vi "ImagerForFlowbit2.vi"() -> ()   [LabVIEW 2011]
uses:
  <vilib>/vision/Image Controls.llb/IMAQ Image.ctl
  <vilib>/Platform/TimedLoop/XDataNode/timing_clust.ctl
  <vilib>/Platform/TimedLoop/XDataNode/nitl_modes.ctl
  <vilib>/Platform/TimedLoop/XDataNode/wakeup.ctl
  <vilib>/Analysis/1siggen.llb/Riffle Array (I32).vi
  <vilib>/Platform/TimedLoop/XDataNode/XDataNode.xnode
  <vilib>/Analysis/NI_AALBase.lvlib
  <vilib>/vision/NI_Vision_Development_Module.lvlib
  <vilib>/Platform/TimedLoop/XDataNode/XDNodeRunTimeDep.lvlib
panel:
  out "队列输出":refnum<queue>
  out "OnlineMap Array":T1[](array[typedef])
  out "DR/R array":T1[](array[typedef])
  out "停止循环":bool
  in  "Stimuli":i32=5
  in  "FrameHeight":i32=576
  in  "FrameWidth":i32=704
  in  "选项卡控件":enum32{"前面板", "参数设置", "OnLineMap"}(tab)
  out "log":string
  out "Stim_ID":i32(listbox)=1
  in  "开始/暂停":bool=TRUE
  in  "停止":bool
  out "重排的 Stim ID":i32[](array[numeric]) caption="重排的{X}"
  out "重排的 Stim ID Index":i32[](array[numeric]) caption="重排的索引"
  out "block":i32
  out "队列中元素数量":i32
  out "Image 2":T1(plugin-control)
  in  "热图":bool
  out "循环持续时间":i64
  out "Recording":bool
  in  "FramesPerStim(100Hz)":i32=16
  in  "Blk目录":path=path "D:/Expt/test"
  in  "文件名":string="G4_E05"
  in  "TimeForPrepare(ms)":u32=1000
  in  "stim ID":u8[](array[numeric])=[0, 2, 4, 6, 8]
  in  "blk总数":i32=500
  in  "stim protocol":T2(array[ring])=[enum."prep stim", enum."wait respirator", enum."show stim", enum."recording data", enum."Blank stim", enum."write data", enum."DR/R", enum."ISI"]
  in  "blank stim":u8
  in  "wait（ms）":u32=10
  in  "ISI（ms）":u32=8000
  in  "FrameBin":i32=25
  in  "datatype":u16(ring)=13 items=["U8"=11, "I16"=12, "U32"=13, "SGL"=14]
  in  "OnlineMap":cluster{"数组 1":i32[], "数组 2":i32[]}[](array[cluster])=[{"数组 1"=[2], "数组 2"=[6]}, {"数组 1"=[4], "数组 2"=[8]}, {"数组 1"=[2, 6], "数组 2"=[4, 8]}, {"数组 1"=[2, 4, 6, 8], "数组 2"=[0]}, {"数组 1"=[2, 4], "数组 2"=[6, 8]}]
  in  "DR/R parameter":T3={"frame_zero_0"=0, "frame_zero_1"=1, "frame_0"=3, "frame_1"=15}
  # "÷"
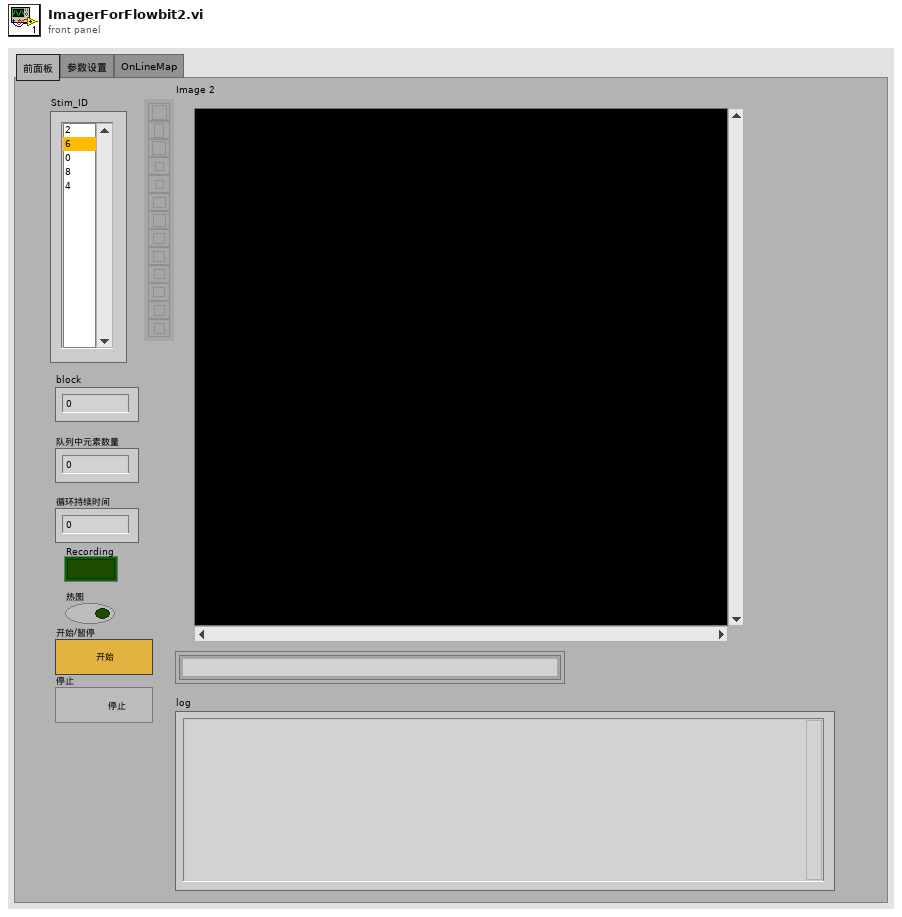
[diagram p1: front panel]
types:
  T1 = typedef "IMAQ Image.ctl" = refnum<image>
  T2 = enum16{"wait", "prep stim", "show stim", "wait respirator", "recording data", "write data", "Blank stim", "wait heart", "ISI", "DR/R", "wait calibrate"}[]
  T3 = cluster{"frame_zero_0":i32, "frame_zero_1":i32, "frame_0":i32, "frame_1":i32}
  T4 = typedef "Image Type" = u32
  T5 = enum16{"Disable External Trigger", "Enable External Trigger"}
  T6 = enum32{"Auto Detect", "RoadRunner", "Raven", "R64"}
  T7 = enum16{"open", "replace", "create", "open or create", "replace or create", "replace or create with confirmation"}
  T8 = enum16{"big-endian, network order", "native, host order", "little-endian"}
  T9 = cluster{"Mean Value":sgl, "Standard Variation":sgl, "Minimal Value":sgl, "Maximal Value":sgl, "Area (calibrated)":sgl, "Area (pixels)":u32, "%":sgl, "Calibration Valid":bool}
  T10 = typedef "XDNodeRunTimeDep.lvlib/timing_clust.ctl" = cluster{"Expected End [f-1]":u64, "Actual End [f-1]":u64, "Finished Late? [f-1]":bool, "Expected End [i-1]":u64, "Actual End [i-1]":u64, "Finished Late? [i-1]":bool, "Expected Start [i]":u64, "Actual Start [i]":u64, "Expected Start [f]":u64, "Actual Start [f]":u64, "Source Name":string, "Structure Name":string, "Period":i64, "Deadline":i64, "Offset":i64, "Start":i64, "Priority":i32, "Timeout":i32, "Mode":T11, "Wakeup Reason":T12, "Error":errorcluster, "Source Type":string, "Secondary Source Type":string, "Global End Time":u64, "Global Start Time":u64, "Frame Duration":u64, "Iteration Duration":u64, "Assigned CPU":i32, "I/O Scan Engine Mode":u32}
  T11 = typedef "XDNodeRunTimeDep.lvlib/nitl_modes.ctl" = enum32{"No Change", "Process missed periods, maintain original phase", "Discard missed periods, maintain original phase", "Process missed periods, ignore original phase", "Discard missed periods, ignore original phase"}
  T12 = typedef "XDNodeRunTimeDep.lvlib/wakeup.ctl" = enum32{"Normal", "Aborted", "Asynchronous wakeup", "Timing source error", "Timed loop error", "Timeout"}
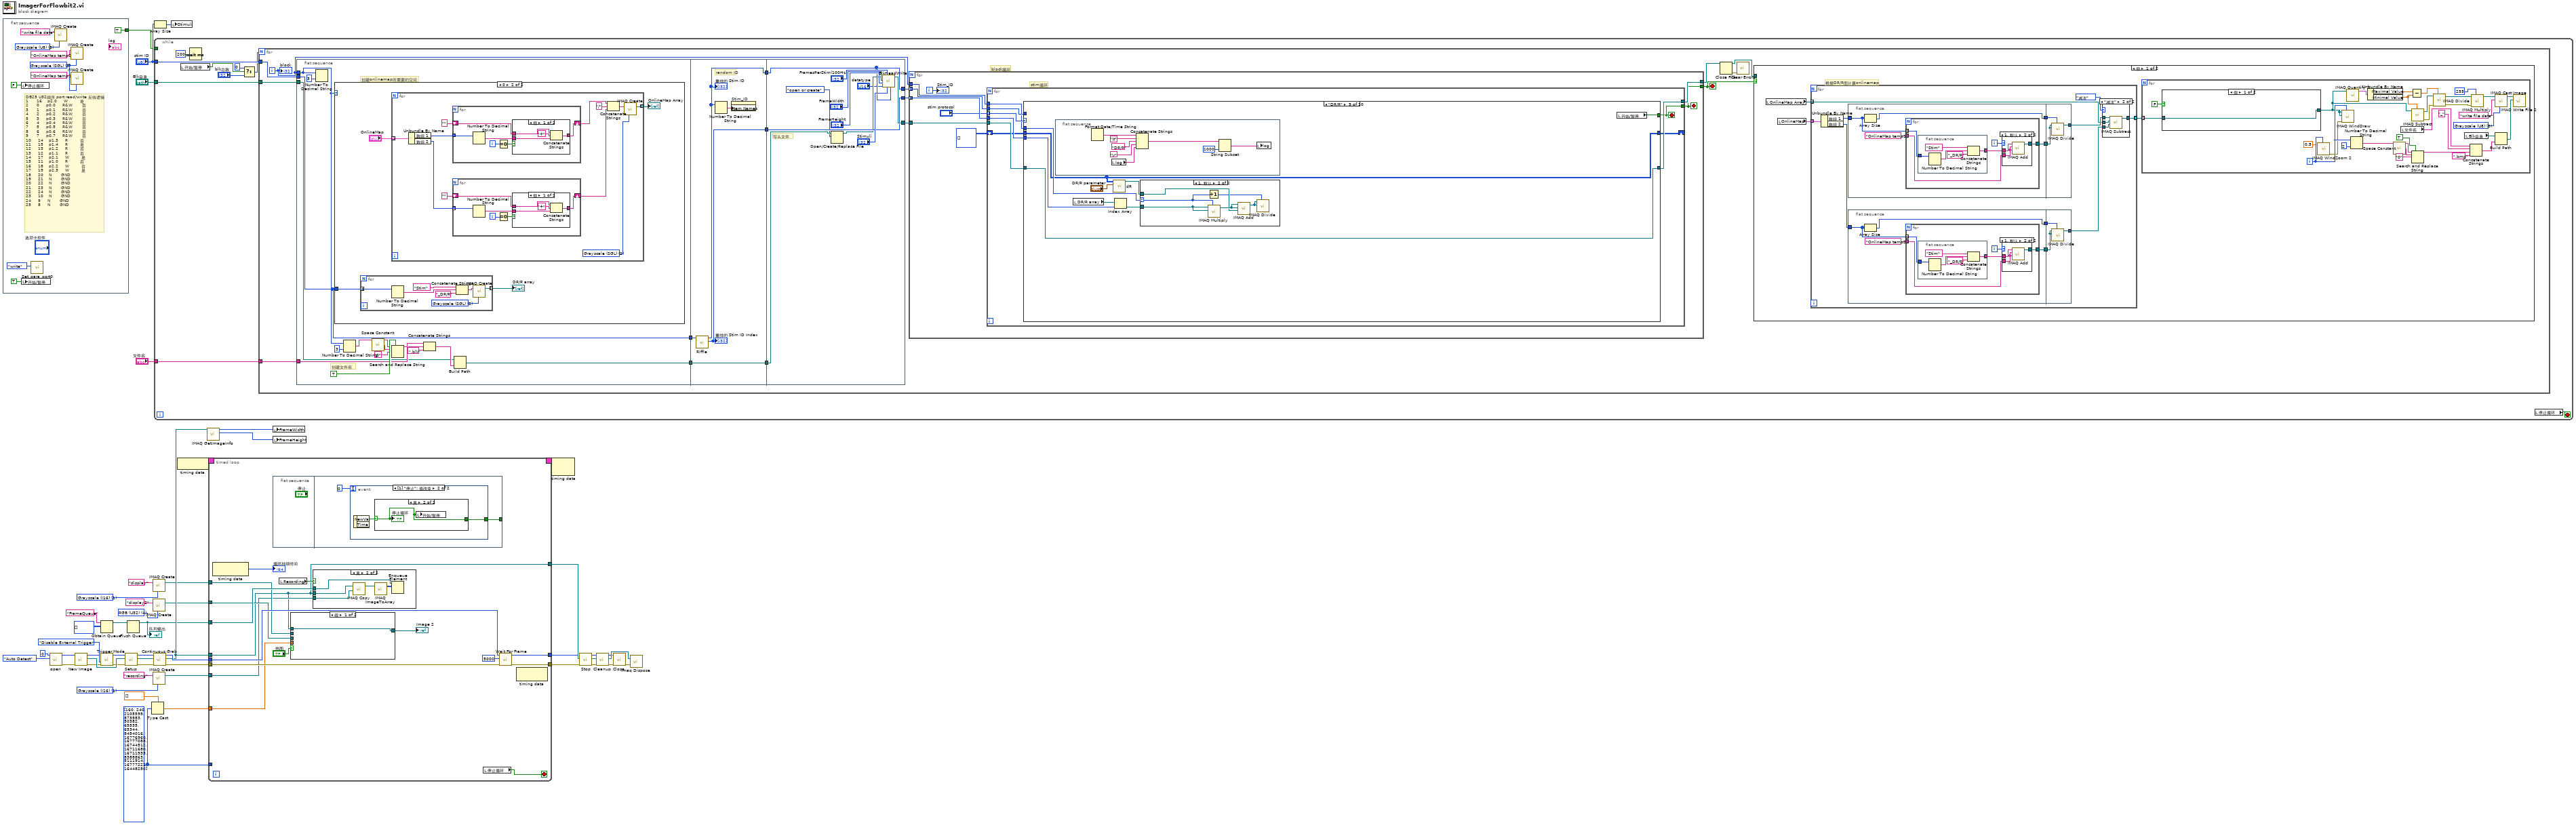
[diagram p0: block diagram]
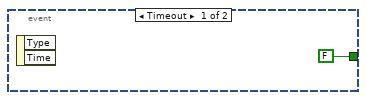
[diagram p2: hidden frame]
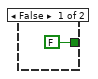
[diagram p3: hidden frame]
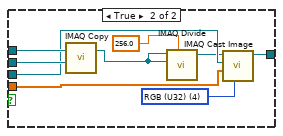
[diagram p4: hidden frame]
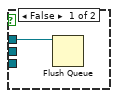
[diagram p5: hidden frame]
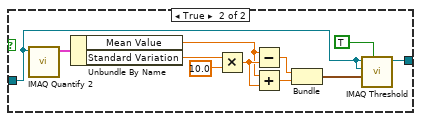
[diagram p6: hidden frame]
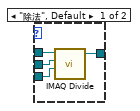
[diagram p7: hidden frame]
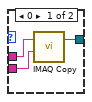
[diagram p8: hidden frame]
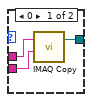
[diagram p9: hidden frame]
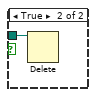
[diagram p10: hidden frame]
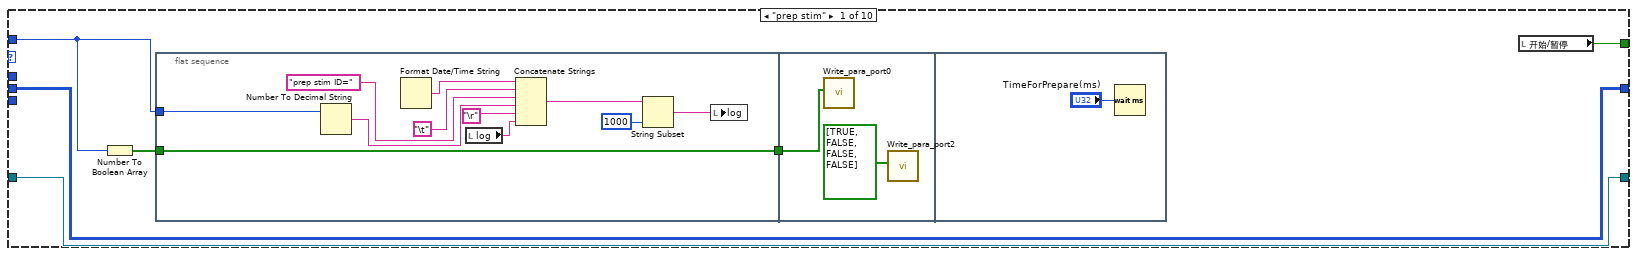
[diagram p14: hidden frame]
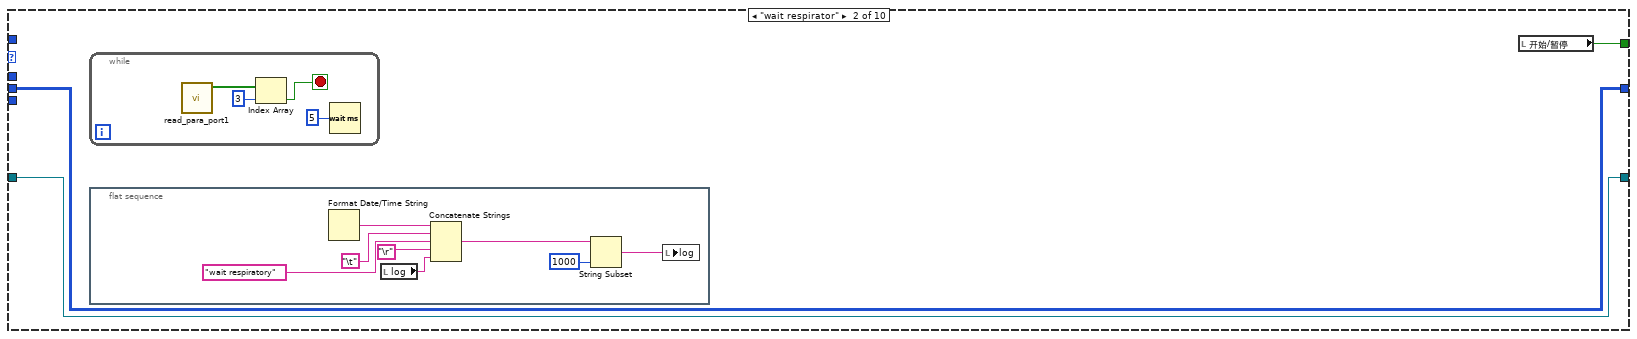
[diagram p15: hidden frame]
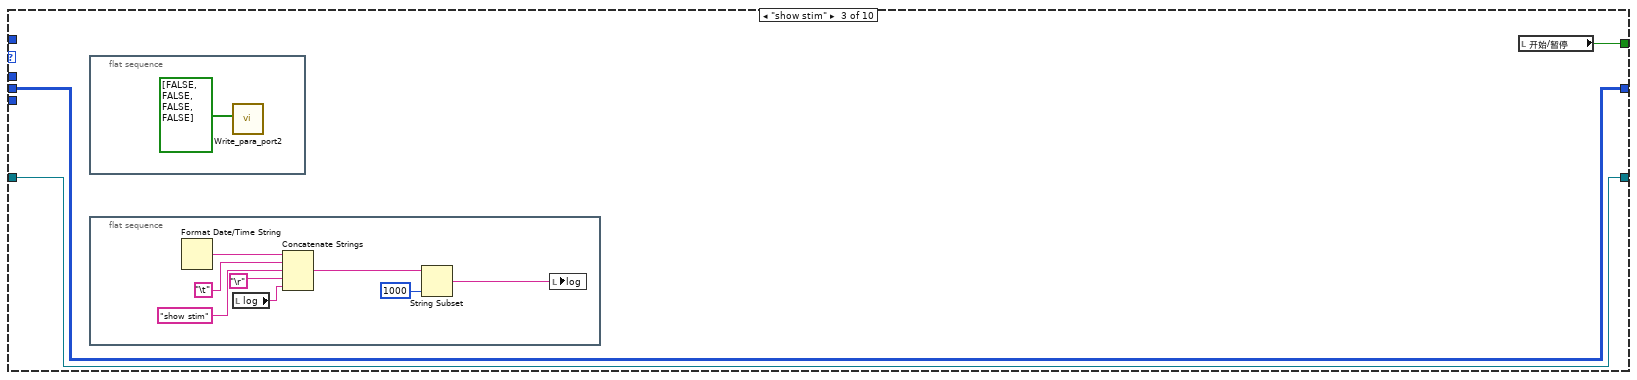
[diagram p16: hidden frame]
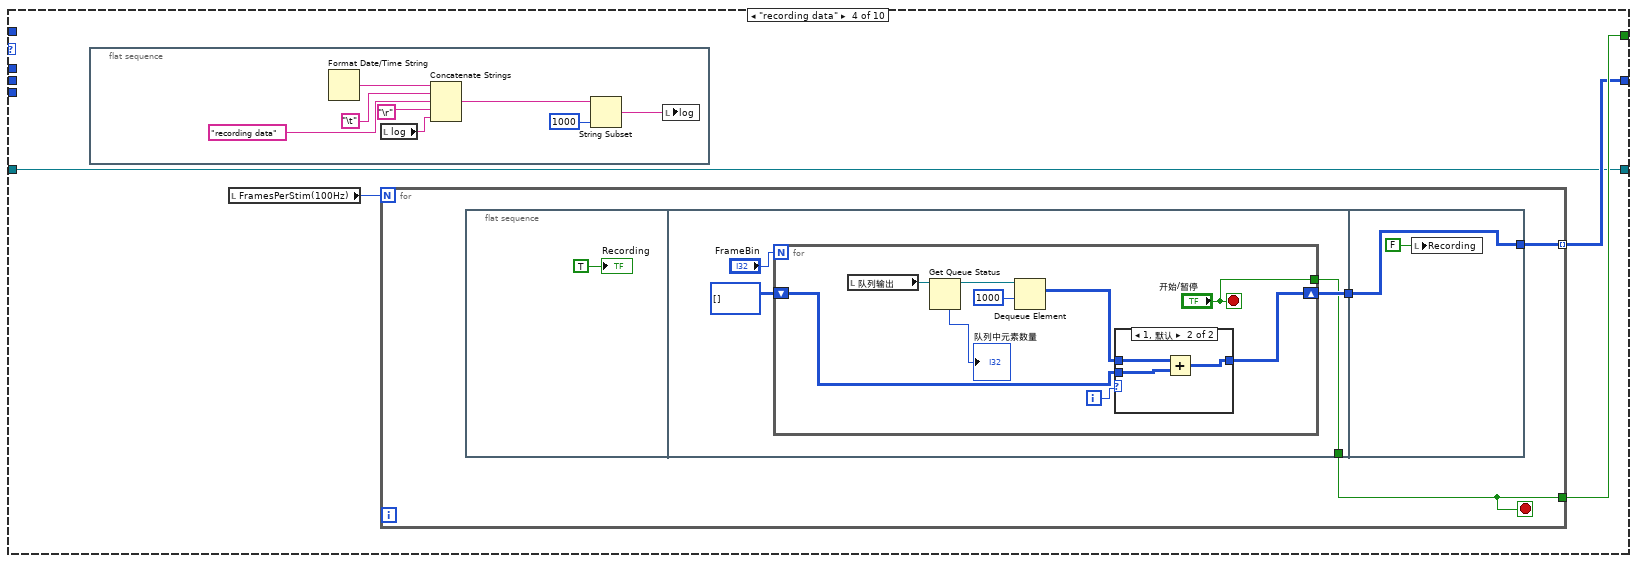
[diagram p17: hidden frame]
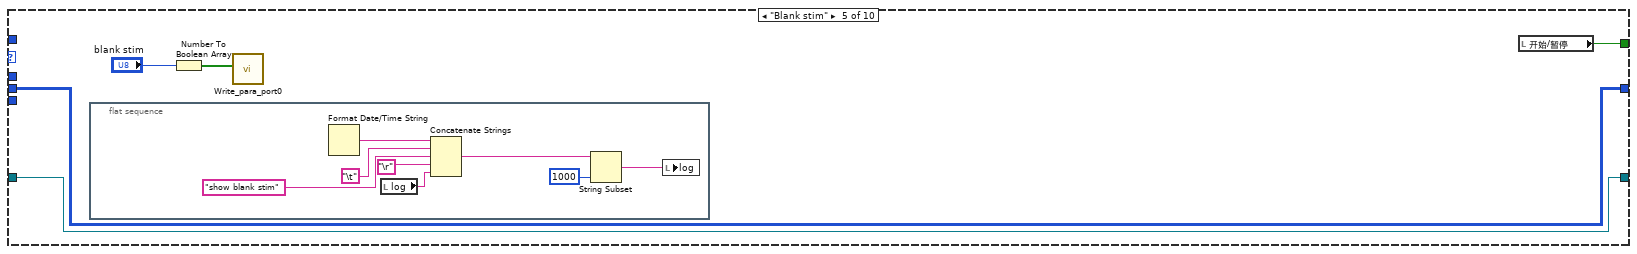
[diagram p19: hidden frame]
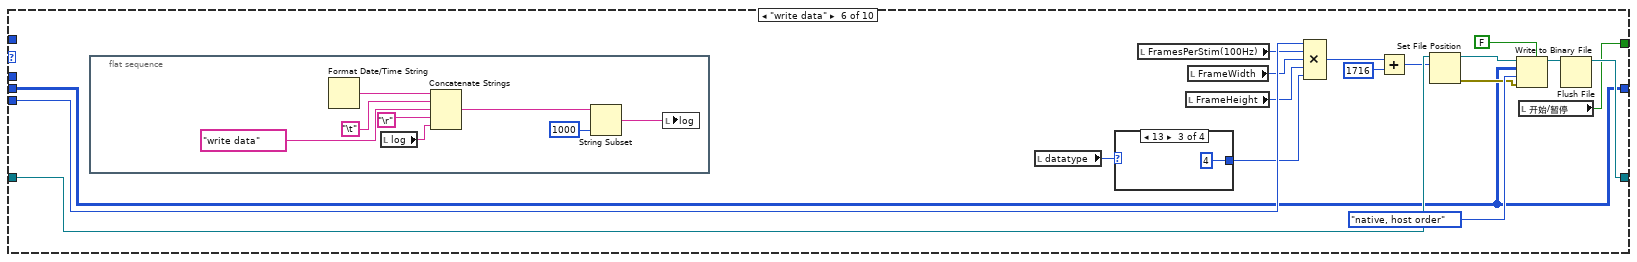
[diagram p20: hidden frame]
diagram:
  w12 = T4 4 items=["Grayscale (U8)", "Grayscale (I16)", "Grayscale (SGL)", "Complex (CSG)", "RGB (U32)", "HSL (U32)", "RGB (U64)", "Grayscale (U16)"] ("Image Type")
  w10 = u32[] [160, 240, 2105599, 873983, 50382, 65535, 65344, 8454016, 16776960, 16777088, 16744512, 16711680, 16711935, 8388863, 5111914, 16777222, 16448250] ("数组")
  w16 = T4 1 items=["Grayscale (U8)", "Grayscale (I16)", "Grayscale (SGL)", "Complex (CSG)", "RGB (U32)", "HSL (U32)", "RGB (U64)", "Grayscale (U16)"] ("Image Type")
  w18 = T4 1 items=["Grayscale (U8)", "Grayscale (I16)", "Grayscale (SGL)", "Complex (CSG)", "RGB (U32)", "HSL (U32)", "RGB (U64)", "Grayscale (U16)"] ("Image Type")
  n1 = flat-sequence {
    tunnel: [TRUE ("Zoom to Fit Mode")] -> w1
    frame #0 {
      w53 = T4 0 items=["Grayscale (U8)", "Grayscale (I16)", "Grayscale (SGL)", "Complex (CSG)", "RGB (U32)", "HSL (U32)", "RGB (U64)", "Grayscale (U16)"] ("Image Type")
      w56 = T4 2 items=["Grayscale (U8)", "Grayscale (I16)", "Grayscale (SGL)", "Complex (CSG)", "RGB (U32)", "HSL (U32)", "RGB (U64)", "Grayscale (U16)"] ("Image Type")
      # "DB25\tU32顺序\tport\tread/write\t反转逻辑\n1\t     16\t   p2.0    \tW\t        是\n2\t     0    \tp0.0\t   \tR&W\t      否\n3\t     1\t\t   p0.1\t   \tR&W      \t否\n4\t\t    2\t   \tp0.2   \t\tR&W      \t否\n5\t\t    3\t\t   p0.3   \t\tR&W\t      否\n6\t\t    4\t   \tp0.4   \t\tR&W      \t否\n7\t\t    5\t   \tp0.5   \t\tR&W      \t否\n8\t\t    6\t   \tp0.6\t   \tR&W      \t否\n9\t    \t7\t   \tp0.7\t   \tR&W\t      否\n10\t    14   \tp1.3   \t\tR        \t否\n11\t   \t15   \tp1.4   \t\tR        \t是\n12\t   \t13   \tp1.2\t   \tR        \t否\n13    \t12   \tp1.1\t   \tR        \t否\n14     17   \tp2.1\t   \tW        \t是\n15    \t11   \tp1.0   \t\tR\t        否\n16    \t18   \tp2.2   \t\tW        \t否\n17    \t19\t   p2.3   \t\tW\t        是\n18    \t20   \tN   \t  \tGND\t\n19    \t21   \tN   \t  \tGND\t\n20\t    22\t   N\t  \t  \tGND\t\n21\t    23\t   N  \t  \t\tGND\t\n22\t    24\t   N  \t  \t\tGND\t\n23    \t10   \tN  \t  \t\tGND\t\n24    \t9\t    N  \t  \t\tGND\t\n25\t    8    \tN  \t  \t\tGND"
      n2 = local write "停止循环"(FALSE ("开始/暂停")) -> ()
      n3 = local write "开始/暂停"(TRUE ("开始/暂停")) -> ()
      n4 = call "Set_para_port0.vi"("R or W"=enum16{"read", "write"}."write") -> ()  [unwired: 9 in, 2 out]
      n5 = call "IMAQ Create"("Image Name"="write file data", "Image Type"=w53) -> ()  [unwired: 3 in, 2 out]
      n6 = call "IMAQ Create"("Image Name"="OnlineMap temp2", "Image Type"=w56) -> ()  [unwired: 3 in, 2 out]
      n7 = call "IMAQ Create"("Image Name"="OnlineMap temp1", "Image Type"=w56) -> ()  [unwired: 3 in, 2 out]
    }
  }
  n8 = call <vilib>:"open.vi"("Board Type"=T6."Auto Detect", "Board Number"=u32 0) -> ("error out"=w34:errorcluster, "RefBrdOut"=w29:u32)  [unwired: 2 in, 5 out]
  n9 = call <vilib>:"New Image.vi"("RefBrdIn"=w29, "error in"=w34) -> ("RefBrdOut"=w28:u32, "Image"=w43:T1, "error out"=w35:errorcluster)  [unwired: 6 in]
  n10 = Obtain Queue(name (unnamed)="FrameQueue" ("名称（未命名）"), element data type=i16[][] []) -> (queue out=w5:refnum<queue>)  [unwired: 3 in, 2 out]
  n11 = call <vilib>:"Trigger Mode.vi"("RefBrdIn"=w28, "Trigger Mode"=T5."Disable External Trigger", "error in (no error)"=w35) -> ("RefBrdOut"=w27:u32, "error out"=w36:errorcluster)  [unwired: 6 in]
  n12 = call <vilib>:"Setup.vi"("error in"=w36, "Image In"=w43, "RefBrdIn"=w27) -> ("error out"=w31:errorcluster, "Image"=w32:T1, "RefBrdOut"=w26:u32)  [unwired: 6 in]
  n13 = Flush Queue(queue=w5) -> (queue out=w4:refnum<queue>)  [unwired: 1 in, 2 out]
  "队列输出" <- w4
  n14 = Type Cast(type=sgl[] [] ("单精度浮点"), x=w10) -> (*(type *) &x=w8:sgl[])
  n15 = call "IMAQ Create"("Image Name"="display", "Image Type"=w16) -> ("New Image"=w14:T1)  [unwired: 3 in, 1 out]
  n16 = call "IMAQ Create"("Image Name"="display2", "Image Type"=w12) -> ("New Image"=w11:T1)  [unwired: 3 in, 1 out]
  n17 = call "IMAQ Create"("Image Name"="recording", "Image Type"=w18) -> ("New Image"=w20:T1)  [unwired: 3 in, 1 out]
  n18 = call <vilib>:"Continuous Grab.vi"("error in (no error)"=w31, "Image In"=w32, "RefBrdIn"=w26) -> ("error out"=w30:errorcluster, "Image"=w17:T1, "RefBrdOut"=w25:u32)  [unwired: 6 in]
  n19 = Array Size(array="stim ID") -> (size(s)=w49:i32)
  n20 = while {
    tunnel: "stim ID" -> [w69]
    tunnel: "文件名" -> [w68]
    tunnel: "Blk目录" -> [w67]
    tunnel: w1 -> [_]
    stop <- w65 stop-if-true
    n21 = local read "开始/暂停"() -> (w64:bool)
    n22 = Wait (ms)(milliseconds to wait=u32 200 ("等待时间（毫秒）")) -> ()  [unwired: 1 out]
    n23 = Select(t=0, s=w64, f="blk总数") -> (s? t:f=w61:i32)
    n24 = for {
      N: w61 -> [_]
      tunnel: w69 -> [w73]
      tunnel: w68 -> [w85]
      tunnel: w67 -> [w84]
      i -> [w74]
      stop <- w76 stop-if-true
      # "block循环"
      n25 = flat-sequence {
        tunnel: [w201] -> w82
        tunnel: [w200] -> w72
        tunnel: w74 -> [w199]
        tunnel: w85 -> [w206]
        tunnel: w84 -> [w202]
        tunnel: w73 -> [w200]
        tunnel: w82 -> [w261]
        tunnel: [w261] -> w81
        tunnel: [w259] -> w80
        tunnel: w72 -> [w258]
        tunnel: [w257] -> w71
        tunnel: w81 -> [w265]
        tunnel: [w268] -> w83
        tunnel: w80 -> [w267]
        tunnel: [w267] -> w79
        tunnel: w71 -> [w266]
        tunnel: [w266] -> w70
        frame #0 {
          # "创建onlinemap所需要的空间"
          # "创建文件名"
          n26 = Number To Decimal String(number=w199, width (-)=i16 3 ("宽度(-)")) -> ()  [unwired: 1 out]
          n27 = case shown="0" w199 {
            tunnel: w200 -> [_ w216]
            frame 1, Default {
            }
            frame 0 {
              n28 = for {
                tunnel: w216 -> [w253] mode=indexing
                tunnel: [w250] -> w215 mode=indexing
                w256 = T4 2 items=["Grayscale (U8)", "Grayscale (I16)", "Grayscale (SGL)", "Complex (CSG)", "RGB (U32)", "HSL (U32)", "RGB (U64)", "Grayscale (U16)"] ("Image Type")
                n29 = Number To Decimal String(number=w253) -> (decimal integer string=w254:string)  [unwired: 1 in]
                n30 = Concatenate Strings("Stim", w254, "_DR/R" ("字符串")) -> (w251:string)
                n31 = call "IMAQ Create"("Image Name"=w251, "Image Type"=w256) -> ("New Image"=w250:T1)  [unwired: 3 in, 1 out]
              }
              "DR/R array" <- w215
              n32 = for {
                tunnel: "OnlineMap" -> [w227] mode=indexing
                tunnel: [w217] -> w213 mode=indexing
                w225 = T4 2 items=["Grayscale (U8)", "Grayscale (I16)", "Grayscale (SGL)", "Complex (CSG)", "RGB (U32)", "HSL (U32)", "RGB (U64)", "Grayscale (U16)"] ("Image Type")
                n33 = Unbundle By Name(w227) -> ("数组 1"=w226:i32[], "数组 2"=w222:i32[])
                n34 = for {
                  tunnel: w226 -> [w242] mode=indexing
                  shift-right: [w240] -> w223
                  shift-left: "" -> [w239]
                  i -> [w244]
                  n35 = Number To Decimal String(number=w242) -> (decimal integer string=w241:string)  [unwired: 1 in]
                  n36 = Equal To 0?(x=w244) -> (x = 0?=w243:bool)
                  n37 = case shown="假" w243 {
                    tunnel: w241 -> [w245 w249]
                    tunnel: [w248 w249] -> w240
                    tunnel: w239 -> [w247 _]
                    frame False {
                      n38 = Concatenate Strings(w247, "+" ("字符串"), w245) -> (w248:string)
                    }
                    frame True {
                    }
                  }
                }
                n39 = for {
                  tunnel: w222 -> [w231] mode=indexing
                  shift-right: [w229] -> w220
                  shift-left: "" -> [w228]
                  i -> [w233]
                  n40 = Number To Decimal String(number=w231) -> (decimal integer string=w230:string)  [unwired: 1 in]
                  n41 = Equal To 0?(x=w233) -> (x = 0?=w232:bool)
                  n42 = case shown="假" w232 {
                    tunnel: w230 -> [w234 w238]
                    tunnel: [w237 w238] -> w229
                    tunnel: w228 -> [w236 _]
                    frame False {
                      n43 = Concatenate Strings(w236, "+" ("字符串"), w234) -> (w237:string)
                    }
                    frame True {
                    }
                  }
                }
                n44 = Concatenate Strings(w223, "/" ("字符串"), w220) -> (w218:string)
                n45 = call "IMAQ Create"("Image Name"=w218, "Image Type"=w225) -> ("New Image"=w217:T1)  [unwired: 3 in, 1 out]
              }
              "OnlineMap Array" <- w213
            }
          }
          n46 = Number To Decimal String(number=w199, width (-)=i16 3 ("宽度(-)")) -> (decimal integer string=w208:string)
          n47 = call <vilib>:"Space Constant.vi"() -> ("String"=w209:string)
          n48 = Search and Replace String(replace all?=TRUE ("替换全部？(F)"), input string=w208, search string=w209, replace string="0" ("替换字符串(\"\")")) -> (result string=w205:string)  [unwired: 4 in, 3 out]
          n49 = Concatenate Strings(w206, w205, ".blk" ("字符串")) -> (w203:string)
          n50 = Build Path(base path=w202, name or relative path=w203) -> (appended path=w201:path)
        }
        frame #1 {
          # "random ID"
          n51 = call-poly <vilib>:"Riffle.vi"("X"=w258) -> ("Riffled Index"=w257:i32[], "Riffled {X}"=w259:i32[])  [unwired: 8 in, 1 out]
          "重排的 Stim ID Index" <- w257
          "重排的 Stim ID" <- w259
          n52 = Number To Decimal String(number=w259) -> (decimal integer string=w260:string[])  [unwired: 1 in]
          n53 = property on="Stim_ID" class="LstBox (严格)"("Item Names"=w260) -> ()  [unwired: 2 in, 2 out]
        }
        frame #2 {
          # "写头文件"
          n54 = Open/Create/Replace File(file path (use dialog)=w265, operation (0:open)=T7."open or create" ("操作(0:open)")) -> (refnum out=w263:refnum<file>)  [unwired: 4 in, 2 out]
          n55 = call "BlkHeadWrite.vi"("SequenceOfID"=w267, "Stimuli"="Stimuli", "FramesPerStim"="FramesPerStim(100Hz)", "datatype"="datatype", "FrameHeight"="FrameHeight", "FrameWidth"="FrameWidth", "BlkFile"=w263) -> ("引用句柄输出"=w268:refnum<file>)  [unwired: 4 in]
        }
      }
      n56 = for {
        tunnel: w83 -> [w281]
        tunnel: [w279] -> w77
        tunnel: w70 -> [w280] mode=indexing
        tunnel: w79 -> [w278] mode=indexing
        tunnel: [w277] -> w76
        tunnel: w74 -> [w273]
        i -> [w276]
        stop <- w277 stop-if-true
        # "stim循环"
        n57 = for {
          tunnel: w280 -> [w289]
          tunnel: w278 -> [w287]
          tunnel: [w283] -> w277
          shift-right: [w286] -> _
          shift-left: u32[][][] [] ("初始化的数组") -> [w285]
          tunnel: "stim protocol" -> [w284] mode=indexing
          tunnel: w281 -> [w290]
          tunnel: [w288] -> w279
          tunnel: w273 -> [w282]
          stop <- w283 stop-if-true
          n58 = case shown="\"DR/R\"" w284 {
            tunnel: w290 -> [w293 w311 w326 w338 w373 w403 w417 w432 w452 w470]
            tunnel: w289 -> [_ _ _ _ _ w402 _ _ w450 _]
            tunnel: [w293 w311 w326 w338 w373 w390 w417 w432 w452 w470] -> w288
            tunnel: w287 -> [w291 _ _ _ _ _ _ _ _ _]
            tunnel: [w294 w312 w327 w340 w374 w388 w418 w433 w451 w471] -> w283
            tunnel: [w295 w313 w328 w339 w375 w389 w419 w434 w445 w472] -> w286
            tunnel: w285 -> [w295 w313 w328 _ w375 w389 w419 w434 w445 w472]
            tunnel: w282 -> [_ _ _ _ _ _ _ _ w449 _]
            frame "prep stim" {
              n59 = Number To Boolean Array(number=w291) -> (Boolean array=w296:bool[])
              n60 = flat-sequence {
                tunnel: w296 -> [w307]
                tunnel: [w307] -> w292
                tunnel: w291 -> [w306]
                tunnel: w292 -> [w309]
                frame #0 {
                  n61 = Number To Decimal String(number=w306) -> (decimal integer string=w303:string)  [unwired: 1 in]
                  n62 = Format Date/Time String() -> (date/time string=w305:string)  [unwired: 3 in]
                  n63 = local read "log"() -> (w299:string)
                  n64 = Concatenate Strings(w305, "\t", "prep stim ID=" ("字符串"), w303, "\r", w299) -> (w301:string)
                  n65 = String Subset(string=w301, length (rest)=1000 ("y")) -> (substring=w300:string)  [unwired: 1 in]
                  n66 = local write "log"(w300) -> ()
                }
                frame #1 {
                  n67 = call "Write_para_port0.vi"("port0（8元素）"=w309) -> ()  [unwired: 10 in, 1 out]
                  n68 = call "Write_para_port2.vi"("port2（4元素）"=bool[] [TRUE, FALSE, FALSE, FALSE] ("port2")) -> ()  [unwired: 10 in, 1 out]
                }
                frame #2 {
                  n69 = Wait (ms)(milliseconds to wait="TimeForPrepare(ms)") -> ()  [unwired: 1 out]
                }
              }
              n70 = local read "开始/暂停"() -> (w294:bool)
            }
            frame "wait respirator" {
              n71 = while {
                stop <- w323 stop-if-true
                n72 = call "read_para_port1.vi"() -> ("port1（5元素）"=w325:bool[])  [unwired: 10 in, 1 out]
                n73 = Index Array(array=w325, index=3 ("索引")) -> (element=w323:bool)
                n74 = Wait (ms)(milliseconds to wait=u32 5 ("等待时间（毫秒）")) -> ()  [unwired: 1 out]
              }
              n75 = flat-sequence {
                frame #0 {
                  n76 = Format Date/Time String() -> (date/time string=w321:string)  [unwired: 3 in]
                  n77 = local read "log"() -> (w316:string)
                  n78 = Concatenate Strings(w321, "\t", "wait respiratory" ("字符串"), "\r", w316) -> (w318:string)
                  n79 = String Subset(string=w318, length (rest)=1000 ("y")) -> (substring=w317:string)  [unwired: 1 in]
                  n80 = local write "log"(w317) -> ()
                }
              }
              n81 = local read "开始/暂停"() -> (w312:bool)
            }
            frame "show stim" {
              n82 = flat-sequence {
                frame #0 {
                  n83 = call "Write_para_port2.vi"("port2（4元素）"=bool[] [FALSE, FALSE, FALSE, FALSE] ("port2")) -> ()  [unwired: 10 in, 1 out]
                }
              }
              n84 = flat-sequence {
                frame #0 {
                  n85 = Format Date/Time String() -> (date/time string=w336:string)  [unwired: 3 in]
                  n86 = local read "log"() -> (w331:string)
                  n87 = Concatenate Strings(w336, "\t", "show stim" ("字符串"), "\r", w331) -> (w333:string)
                  n88 = String Subset(string=w333, length (rest)=1000 ("y")) -> (substring=w332:string)  [unwired: 1 in]
                  n89 = local write "log"(w332) -> ()
                }
              }
              n90 = local read "开始/暂停"() -> (w327:bool)
            }
            frame "recording data" {
              n91 = flat-sequence {
                frame #0 {
                  n92 = Format Date/Time String() -> (date/time string=w349:string)  [unwired: 3 in]
                  n93 = local read "log"() -> (w344:string)
                  n94 = Concatenate Strings(w349, "\t", "recording data" ("字符串"), "\r", w344) -> (w346:string)
                  n95 = String Subset(string=w346, length (rest)=1000 ("y")) -> (substring=w345:string)  [unwired: 1 in]
                  n96 = local write "log"(w345) -> ()
                }
              }
              n97 = local read "FramesPerStim(100Hz)"() -> (w341:i32)
              n98 = for {
                N: w341 -> [_]
                tunnel: [w350] -> w339 mode=indexing
                tunnel: [w352] -> w340
                stop <- w352 stop-if-true
                n99 = flat-sequence {
                  tunnel: [w354] -> w352
                  tunnel: [w356] -> w351
                  tunnel: [w372] -> w350
                  tunnel: w351 -> [w372]
                  frame #0 {
                    "Recording" <- TRUE ("Recording")
                  }
                  frame #1 {
                    n100 = for {
                      N: "FrameBin" -> [_]
                      shift-right: [w365] -> w356
                      shift-left: u32[][] [] ("初始化的数组") -> [w366]
                      tunnel: ["开始/暂停"] -> w354
                      i -> [w364]
                      stop <- "开始/暂停" stop-if-true
                      n101 = local read "队列输出"() -> (w362:refnum<queue>)
                      n102 = Get Queue Status(queue=w362) -> (queue out=w360:refnum<queue>, # elements in queue=→"队列中元素数量":i32)  [unwired: 2 in, 6 out]
                      n103 = Dequeue Element(queue=w360, timeout in ms (-1)=1000 ("超时毫秒(-1)")) -> (element=w359:i16[][])  [unwired: 1 in, 3 out]
                      n104 = case shown="1, 默认" w364 {
                        tunnel: w359 -> [w367 w370]
                        tunnel: w366 -> [_ w369]
                        tunnel: [w367 w368] -> w365
                        frame 0 {
                        }
                        frame 1, Default {
                          n105 = Add(x=w370, y=w369) -> (x+y=w368:u32[][])
                        }
                      }
                    }
                  }
                  frame #2 {
                    n106 = local write "Recording"(FALSE ("Recording")) -> ()
                  }
                }
              }
            }
            frame "Blank stim" {
              n107 = flat-sequence {
                frame #0 {
                  n108 = Format Date/Time String() -> (date/time string=w385:string)  [unwired: 3 in]
                  n109 = local read "log"() -> (w380:string)
                  n110 = Concatenate Strings(w385, "\t", "show blank stim" ("字符串"), "\r", w380) -> (w382:string)
                  n111 = String Subset(string=w382, length (rest)=1000 ("y")) -> (substring=w381:string)  [unwired: 1 in]
                  n112 = local write "log"(w381) -> ()
                }
              }
              n113 = Number To Boolean Array(number="blank stim") -> (Boolean array=w376:bool[])
              n114 = call "Write_para_port0.vi"("port0（8元素）"=w376) -> ()  [unwired: 10 in, 1 out]
              n115 = local read "开始/暂停"() -> (w374:bool)
            }
            frame "write data" {
              n116 = flat-sequence {
                frame #0 {
                  n117 = Format Date/Time String() -> (date/time string=w415:string)  [unwired: 3 in]
                  n118 = local read "log"() -> (w410:string)
                  n119 = Concatenate Strings(w415, "\t", "write data" ("字符串"), "\r", w410) -> (w412:string)
                  n120 = String Subset(string=w412, length (rest)=1000 ("y")) -> (substring=w411:string)  [unwired: 1 in]
                  n121 = local write "log"(w411) -> ()
                }
              }
              n122 = local read "datatype"() -> (w387:u16)
              n123 = case shown="13" w387 {
                tunnel: [1 2 4 4] -> w386
                frame 11, Default {
                }
                frame 12 {
                }
                frame 13 {
                }
                frame 14 {
                }
              }
              n124 = local read "FramesPerStim(100Hz)"() -> (w394:i32)
              n125 = local read "FrameHeight"() -> (w392:i32)
              n126 = local read "FrameWidth"() -> (w393:i32)
              n127 = Compound Arithmetic op=MULTIPLY(w402, w394, w393, w392, w386) -> (w397:i32)
              n128 = Add(x=w397, y=i64 1716 ("偏移量（字节）（0）")) -> (x+y=w395:i64)
              n129 = Set File Position(offset (in bytes) (0)=w395, refnum=w403) -> (refnum out=w400:refnum<file>, error out=w398:errorcluster)  [unwired: 2 in]
              n130 = Write to Binary File(file (use dialog)=w400, data=w389, error in=w398, 5:FALSE ("预置数组或字符串大小？(T)"), 9:T8."native, host order" ("字节顺序(0:big-endian, network order)")) -> (refnum out=w391:refnum<file>)  [unwired: 1 in, 2 out]
              n131 = local read "开始/暂停"() -> (w388:bool)
              n132 = Flush File(refnum=w391) -> (refnum out=w390:refnum<file>)  [unwired: 1 in, 1 out]
            }
            frame "ISI" {
              n133 = flat-sequence {
                tunnel: "ISI（ms）" -> [w423]
                tunnel: "ISI（ms）" -> [w430]
                frame #0 {
                  n134 = Number To Decimal String(number=w423) -> (decimal integer string=w427:string)  [unwired: 1 in]
                  n135 = Format Date/Time String() -> (date/time string=w429:string)  [unwired: 3 in]
                  n136 = local read "log"() -> (w422:string)
                  n137 = Concatenate Strings(w429, "\t", "ISI(ms)=" ("字符串"), w427, "\r", w422) -> (w425:string)
                  n138 = String Subset(string=w425, length (rest)=1000 ("y")) -> (substring=w424:string)  [unwired: 1 in]
                  n139 = local write "log"(w424) -> ()
                }
                frame #1 {
                  n140 = Wait (ms)(milliseconds to wait=w430) -> ()  [unwired: 1 out]
                }
              }
              n141 = local read "开始/暂停"() -> (w418:bool)
            }
            frame "wait", Default {
              n142 = Wait (ms)(milliseconds to wait="wait（ms）") -> ()  [unwired: 1 out]
              n143 = flat-sequence {
                tunnel: "wait（ms）" -> [w438]
                frame #0 {
                  n144 = Number To Decimal String(number=w438) -> (decimal integer string=w442:string)  [unwired: 1 in]
                  n145 = Format Date/Time String() -> (date/time string=w444:string)  [unwired: 3 in]
                  n146 = local read "log"() -> (w437:string)
                  n147 = Concatenate Strings(w444, "\t", "wait(ms)=" ("字符串"), w442, "\r", w437) -> (w440:string)
                  n148 = String Subset(string=w440, length (rest)=1000 ("y")) -> (substring=w439:string)  [unwired: 1 in]
                  n149 = local write "log"(w439) -> ()
                }
              }
              n150 = local read "开始/暂停"() -> (w433:bool)
            }
            frame "DR/R" {
              n151 = flat-sequence {
                frame #0 {
                  n152 = Format Date/Time String() -> (date/time string=w461:string)  [unwired: 3 in]
                  n153 = local read "log"() -> (w456:string)
                  n154 = Concatenate Strings(w461, "\t", "DR/R" ("字符串"), "\r", w456) -> (w458:string)
                  n155 = String Subset(string=w458, length (rest)=1000 ("y")) -> (substring=w457:string)  [unwired: 1 in]
                  n156 = local write "log"(w457) -> ()
                }
              }
              n157 = local read "DR/R array"() -> (w446:T1[])
              n158 = call "dR.vi"("DR/R parameter"="DR/R parameter", "数组"=w445) -> ("Image Dst Out"=w448:T1)  [unwired: 9 in]
              n159 = Index Array(array=w446, index=w450) -> (element=w447:T1)
              n160 = case shown="1, 默认" w449 {
                selector: w449 -> [_ w466]
                tunnel: w448 -> [w463 w467]
                tunnel: w447 -> [w462 w469]
                frame 0 {
                  n161 = call "IMAQ Copy"("Image Dst"=w462, "Image Src"=w463) -> ()  [unwired: 4 in, 2 out]
                }
                frame 1, Default {
                  n162 = Increment(x=w466) -> (x+1=w465:i32)
                  n163 = call "IMAQ Multiply"("Image Src A"=w469, "Constant"=w466, "Image Dst"=w469) -> ("Image Dst Out"=w468:T1)  [unwired: 4 in, 1 out]
                  n164 = call "IMAQ Add"("Image Src A"=w468, "Image Dst"=w468, "Image Src B"=w467) -> ("Image Dst Out"=w464:T1)  [unwired: 4 in, 1 out]
                  n165 = call "IMAQ Divide"("Image Src A"=w464, "Constant"=w465, "Image Dst"=w464) -> ()  [unwired: 4 in, 2 out]
                }
              }
              n166 = local read "开始/暂停"() -> (w451:bool)
            }
            frame "wait heart" {
              n167 = flat-sequence {
                frame #0 {
                  n168 = Format Date/Time String() -> (date/time string=w480:string)  [unwired: 3 in]
                  n169 = local read "log"() -> (w475:string)
                  n170 = Concatenate Strings(w480, "\t", "wait heart" ("字符串"), "\r", w475) -> (w477:string)
                  n171 = String Subset(string=w477, length (rest)=1000 ("y")) -> (substring=w476:string)  [unwired: 1 in]
                  n172 = local write "log"(w476) -> ()
                }
              }
              n173 = local read "开始/暂停"() -> (w471:bool)
            }
          }
        }
        "Stim_ID" <- w276
      }
      n174 = Close File(refnum=w77) -> (path=w75:path, error out=w78:errorcluster)  [unwired: 1 in]
      n175 = call <vilib>:"Clear Errors.vi"("error in (no error)"=w78) -> ()  [unwired: 6 in, 1 out]
      n176 = case shown="假" w76 {
        tunnel: w75 -> [_ w198]
        frame False {
          # "根据DR/R图计算onlinemap"
          n177 = local read "OnlineMap Array"() -> (w87:T1[])
          n178 = local read "OnlineMap"() -> (w88:cluster{"数组 1":i32[], "数组 2":i32[]}[])
          n179 = for {
            tunnel: w88 -> [w143] mode=indexing
            tunnel: w87 -> [w134] mode=indexing
            tunnel: [w132] -> w86 mode=indexing
            n180 = Unbundle By Name(w143) -> ("数组 1"=w142:i32[], "数组 2"=w137:i32[])
            n181 = flat-sequence {
              tunnel: w142 -> [w177]
              tunnel: [w176] -> w141
              tunnel: [w175] -> w140
              tunnel: w141 -> [w196]
              tunnel: w140 -> [w197]
              tunnel: [w195] -> w136
              frame #0 {
                n182 = Array Size(array=w177) -> (size(s)=w175:i32)
                n183 = for {
                  tunnel: w177 -> [w183] mode=indexing
                  tunnel: "OnlineMap temp1" ("Image Name") -> [w181]
                  tunnel: [w179] -> w176
                  i -> [w180]
                  n184 = flat-sequence {
                    tunnel: w183 -> [w192]
                    tunnel: [w190] -> w182
                    frame #0 {
                      n185 = Number To Decimal String(number=w192) -> (decimal integer string=w193:string)  [unwired: 1 in]
                      n186 = Concatenate Strings("Stim", w193, "_DR/R" ("字符串")) -> (w190:string)
                    }
                  }
                  n187 = case shown="1, 默认" w180 {
                    tunnel: w182 -> [w186 w189]
                    tunnel: w181 -> [w185 w188]
                    tunnel: [w184 w187] -> w179
                    frame 0 {
                      n188 = call "IMAQ Copy"("Image Dst"=w185, "Image Src"=w186) -> ("Image Dst Out"=w184:T1)  [unwired: 4 in, 1 out]
                    }
                    frame 1, Default {
                      n189 = call "IMAQ Add"("Image Src A"=w189, "Image Dst"=w188, "Image Src B"=w188) -> ("Image Dst Out"=w187:T1)  [unwired: 4 in, 1 out]
                    }
                  }
                }
              }
              frame #1 {
                n190 = call "IMAQ Divide"("Image Src A"=w196, "Constant"=w197, "Image Dst"=w196) -> ("Image Dst Out"=w195:T1)  [unwired: 4 in, 1 out]
              }
            }
            n191 = flat-sequence {
              tunnel: w137 -> [w154]
              tunnel: [w153] -> w139
              tunnel: [w152] -> w138
              tunnel: w139 -> [w173]
              tunnel: w138 -> [w174]
              tunnel: [w172] -> w135
              frame #0 {
                n192 = Array Size(array=w154) -> (size(s)=w152:i32)
                n193 = for {
                  tunnel: w154 -> [w160] mode=indexing
                  tunnel: "OnlineMap temp2" ("Image Name") -> [w158]
                  tunnel: [w156] -> w153
                  i -> [w157]
                  n194 = flat-sequence {
                    tunnel: w160 -> [w169]
                    tunnel: [w167] -> w159
                    frame #0 {
                      n195 = Number To Decimal String(number=w169) -> (decimal integer string=w170:string)  [unwired: 1 in]
                      n196 = Concatenate Strings("Stim", w170, "_DR/R" ("字符串")) -> (w167:string)
                    }
                  }
                  n197 = case shown="1, 默认" w157 {
                    tunnel: w159 -> [w163 w166]
                    tunnel: w158 -> [w162 w165]
                    tunnel: [w161 w164] -> w156
                    frame 0 {
                      n198 = call "IMAQ Copy"("Image Dst"=w162, "Image Src"=w163) -> ("Image Dst Out"=w161:T1)  [unwired: 4 in, 1 out]
                    }
                    frame 1, Default {
                      n199 = call "IMAQ Add"("Image Src A"=w166, "Image Dst"=w165, "Image Src B"=w165) -> ("Image Dst Out"=w164:T1)  [unwired: 4 in, 1 out]
                    }
                  }
                }
              }
              frame #1 {
                n200 = call "IMAQ Divide"("Image Src A"=w173, "Constant"=w174, "Image Dst"=w173) -> ("Image Dst Out"=w172:T1)  [unwired: 4 in, 1 out]
              }
            }
            n201 = case shown="\"减法\"" enum16{"除法", "减法"}."减法" {
              tunnel: w136 -> [w147 w151]
              tunnel: w135 -> [w146 w150]
              tunnel: w134 -> [w145 w149]
              tunnel: [w144 w148] -> w132
              frame "除法", Default {
                n202 = call "IMAQ Divide"("Image Src A"=w147, "Image Dst"=w145, "Image Src B"=w146) -> ("Image Dst Out"=w144:T1)  [unwired: 4 in, 1 out]
              }
              frame "减法" {
                n203 = call "IMAQ Subtract"("Image Src A"=w151, "Image Dst"=w149, "Image Src B"=w150) -> ("Image Dst Out"=w148:T1)  [unwired: 4 in, 1 out]
              }
            }
          }
          n204 = for {
            tunnel: w86 -> [w119] mode=indexing
            i -> [w117]
            w103 = T4 0 items=["Grayscale (U8)", "Grayscale (I16)", "Grayscale (SGL)", "Complex (CSG)", "RGB (U32)", "HSL (U32)", "RGB (U64)", "Grayscale (U16)"] ("Image Type")
            n205 = case shown="假" FALSE {
              tunnel: [w120 w125] -> w98
              tunnel: w119 -> [w120 w124]
              frame False {
              }
              frame True {
                n206 = call "IMAQ Quantify 2"("Image"=w124) -> ("Global Report"=w131:T9)  [unwired: 8 in, 2 out]
                n207 = Unbundle By Name(w131) -> ("Mean Value"=w123:sgl, "Standard Variation"=w122:sgl)
                n208 = Multiply(x=w122, y=sgl 10.0) -> (x*y=w129:sgl)
                n209 = Subtract(x=w123, y=w129) -> (x-y=w128:sgl)
                n210 = Add(x=w123, y=w129) -> (x+y=w127:sgl)
                n211 = Bundle(w128, w127) -> (w126:cluster{sgl, sgl})  [unwired: 1 in]
                n212 = call "IMAQ Threshold"("Keep/Replace Value (Replace)"=TRUE, "Range"=w126, "Image Dst"=w124, "Image Src"=w124) -> ("Image Dst Out"=w125:T1)  [unwired: 6 in, 1 out]
              }
            }
            n213 = call "IMAQ WindZoom 2"("Window Number (0...15)"=w117, "Zoom Factor"=sgl 0.5) -> ("error out"=w99:errorcluster)  [unwired: 6 in, 3 out]
            n214 = call "IMAQ WindDraw"("Window Number (0...15)"=w117, "error in (no error)"=w99, "Title"=w98, "Image"=w98) -> ()  [unwired: 6 in, 2 out]
            n215 = call "IMAQ Quantify 2"("Image"=w98) -> ("Global Report"=w101:T9)  [unwired: 8 in, 2 out]
            n216 = Number To Decimal String(number=w117, width (-)=i16 2 ("宽度(-)")) -> (decimal integer string=w113:string)
            n217 = Unbundle By Name(w101) -> ("Maximal Value"=w100:sgl, "Minimal Value"=w97:sgl)
            n218 = call <vilib>:"Space Constant.vi"() -> ("String"=w112:string)
            n219 = local read "文件名"() -> (w115:string)
            n220 = Subtract(x=w100, y=w97) -> (x-y=w94:sgl)
            n221 = call "IMAQ Subtract"("Image Src A"=w98, "Constant"=w97) -> ("Image Dst Out"=w95:T1, "error out"=w96:errorcluster)  [unwired: 5 in]
            n222 = Search and Replace String(replace all?=TRUE ("替换全部？(F)"), input string=w113, search string=w112, replace string="0" ("替换字符串(\"\")")) -> (result string=w108:string)  [unwired: 4 in, 3 out]
            n223 = call "IMAQ Divide"("Image Src A"=w95, "Constant"=w94, "error in (no error)"=w96) -> ("Image Dst Out"=w92:T1, "error out"=w93:errorcluster)  [unwired: 4 in]
            n224 = local read "Blk目录"() -> (w106:path)
            n225 = Concatenate Strings(w115, "_" ("字符串"), w108, ".bmp" ("字符串")) -> (w105:string)
            n226 = call "IMAQ Multiply"("Image Src A"=w92, "Constant"=255, "error in (no error)"=w93) -> ("Image Dst Out"=w90:T1)  [unwired: 4 in, 1 out]
            n227 = call "IMAQ Cast Image"("Image Type"=w103, "Image Dst"="write file data" ("替换字符串(\"\")"), "Image Src"=w90) -> ("Image Dst Out"=w102:T1)  [unwired: 7 in, 1 out]
            n228 = Build Path(base path=w106, name or relative path=w105) -> (appended path=w104:path)
            n229 = call-poly "IMAQ Write File 2"("File Path"=w104, "Image"=w102) -> ()  [unwired: 8 in, 2 out]
          }
        }
        frame True {
          n230 = Delete(path (use dialog)=w198) -> ()  [unwired: 4 in, 3 out]
        }
      }
      "block" <- w74
    }
    n231 = local read "停止循环"() -> (w65:bool)
  }
  n232 = local write "Stimuli"(w49) -> ()
  n233 = node-c288() -> (w47:T10)
  n234 = call "IMAQ GetImageInfo"("Image"=w17) -> ("Y Resolution"=w2:i32, "X Resolution"=w3:i32)  [unwired: 3 in, 6 out]
  n235 = timed-loop {
    tunnel: [w481] -> w42
    tunnel: [w496] -> w37
    tunnel: w17 -> [w481]
    tunnel: w30 -> [w495]
    tunnel: w25 -> [w494]
    tunnel: [w493] -> w24
    timing: w47 -> [_]
    timing-out: [_] -> w46
    tunnel: w20 -> [w482]
    tunnel: w4 -> [w491]
    tunnel: w14 -> [w487]
    tunnel: w10 -> [_]
    tunnel: w11 -> [w486]
    tunnel: w8 -> [w485]
    stop <- w488 stop-if-true
    n236 = node-c288() -> (→"循环持续时间":i64)  [unwired: 1 in]
    n237 = flat-sequence {
      tunnel: [w497] -> _
      frame #0 {
      }
      frame #1 {
        n238 = event shown="[1] \"停止\": 值改变" {
          selector: _ -> [_ _]
          dyn-events: _ -> [_ _]
          timeout: 0 -> [_ _]
          tunnel: [FALSE w500] -> w497
          event Timeout {
            n239 = event-data() -> ()  [unwired: 1 in, 2 out]
          }
          event "停止": Value Change {
            n240 = event-data() -> ("NewVal"=w501:bool)  [unwired: 1 in, 1 out]
            n241 = case shown="真" w501 {
              selector: w501 -> [_ w503]
              tunnel: [FALSE w503] -> w500
              frame False {
              }
              frame True {
                n242 = local write "开始/暂停"(w503) -> ()
                "停止循环" <- w503
              }
            }
          }
        }
      }
    }
    n243 = local read "Recording"() -> (w489:bool)
    n244 = case shown="假" "热图" {
      tunnel: w487 -> [_ w512]
      tunnel: w481 -> [w504 w510]
      tunnel: [w504 w509] -> w484
      tunnel: w486 -> [_ w507]
      tunnel: w485 -> [_ w506]
      frame False {
      }
      frame True {
        w508 = T4 4 items=["Grayscale (U8)", "Grayscale (I16)", "Grayscale (SGL)", "Complex (CSG)", "RGB (U32)", "HSL (U32)", "RGB (U64)", "Grayscale (U16)"] ("Image Type")
        n245 = call "IMAQ Copy"("Image Dst"=w512, "Image Src"=w510) -> ("Image Dst Out"=w511:T1)  [unwired: 4 in, 1 out]
        n246 = call "IMAQ Divide"("Image Src A"=w511, "Constant"=sgl 256.0, "Image Dst"=w511) -> ("Image Dst Out"=w505:T1)  [unwired: 4 in, 1 out]
        n247 = call "IMAQ Cast Image"("Image Type"=w508, "Lookup Table"=w506, "Image Dst"=w507, "Image Src"=w505) -> ("Image Dst Out"=w509:T1)  [unwired: 6 in, 1 out]
      }
    }
    "Image 2" <- w484
    n248 = case shown="真" w489 {
      tunnel: w491 -> [w514 w519]
      tunnel: w481 -> [_ w517]
      tunnel: w482 -> [_ w515]
      frame False {
        n249 = Flush Queue(queue=w514) -> ()  [unwired: 1 in, 3 out]
      }
      frame True {
        n250 = call "IMAQ Copy"("Image Dst"=w515, "Image Src"=w517) -> ("Image Dst Out"=w516:T1)  [unwired: 4 in, 1 out]
        n251 = call "IMAQ ImageToArray"("Image"=w516) -> ("Image Pixels (I16)"=w518:i16[][])  [unwired: 3 in, 4 out]
        n252 = Enqueue Element(queue=w519, element=w518) -> ()  [unwired: 2 in, 3 out]
      }
    }
    n253 = local read "停止循环"() -> (w488:bool)
    n254 = call <vilib>:"Wait For Frame.vi"("error in (no error)"=w495, "Timeout (mS)"=u32 5000, "RefBrdIn"=w494) -> ("error out"=w496:errorcluster, "RefBrdOut"=w493:u32)  [unwired: 7 in]
    n255 = node-c288() -> ()  [unwired: 1 in, 1 out]
  }
  n256 = local write "FrameWidth"(w3) -> ()
  n257 = local write "FrameHeight"(w2) -> ()
  n258 = node-c288(w46) -> ()  [unwired: 1 out]
  n259 = call <vilib>:"Stop.vi"("error in (no error)"=w37, "Image In"=w42, "RefBrdIn"=w24) -> ("error out"=w38:errorcluster, "Image"=w41:T1, "RefBrdOut"=w23:u32)  [unwired: 6 in]
  n260 = call <vilib>:"Cleanup.vi"("error in (no error)"=w38, "Image In"=w41, "RefBrdIn"=w23) -> ("error out"=w39:errorcluster, "Image"=w40:T1, "RefBrdOut"=w22:u32)  [unwired: 6 in]
  n261 = call <vilib>:"Close.vi"("error in (no error)"=w39, "RefBrdIn"=w22) -> ("error out"=w21:errorcluster)  [unwired: 8 in, 1 out]
  n262 = call "Imaq Dispose"("Image"=w40, "error in (no error)"=w21) -> ()  [unwired: 4 in, 1 out]
